vi "Get Objects in Range.vi"(8 "error in":errorcluster, 9 "Upper Bound":u16 format="%.0x", 10 "Lower Bound":u16 format="%.0x", 11 "Sorted Object Dictionary in":refnum<class "Sorted Object Dictionary.lvclass">) -> (0 "error out":errorcluster, 2 "Entries":refnum<class "OD Entry.lvclass">[](array[class]), 3 "Sorted Object Dictionary out":refnum<class "Sorted Object Dictionary.lvclass">)   [LabVIEW 2019, in "Electronic Datasheet.lvlib" / "Sorted Object Dictionary.lvclass"]
uses:
  Sorted Object Dictionary.lvclass
  OD Entry/OD Entry.lvclass
  Sorted Object Dictionary.lvclass/Sorted Object Dictionary.ctl
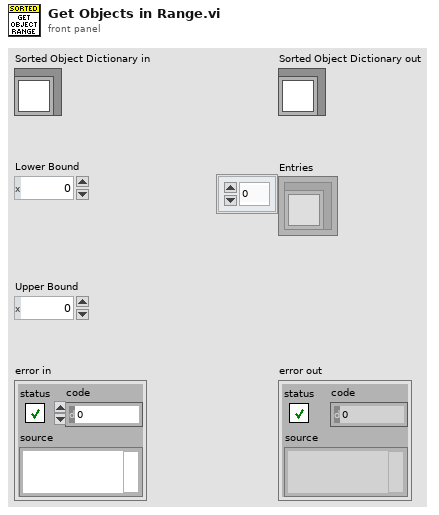
[diagram p1: front panel]
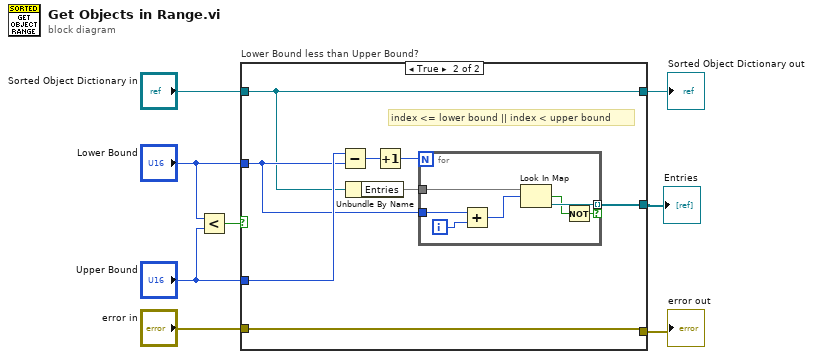
[diagram p0: block diagram]
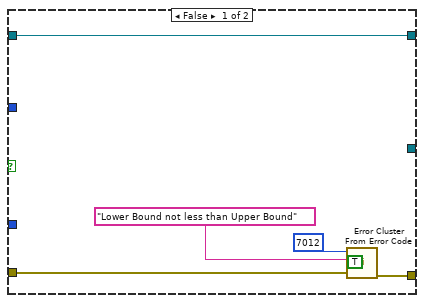
[diagram p2: hidden frame]
diagram:
  n1 = Less?(x="Lower Bound", y="Upper Bound") -> (x < y?=w5:bool)
  n2 = case "Lower Bound less than Upper Bound?" shown="True" w5 {
    tunnel: "Sorted Object Dictionary in" -> [w9 w16]
    tunnel: "Lower Bound" -> [_ w18]
    tunnel: "Upper Bound" -> [_ w21]
    tunnel: "error in" -> [w14 w17]
    tunnel: [w13 w17] -> w3
    tunnel: [w9 w16] -> w2
    tunnel: [_ w15] -> w1
    frame False {
      n3 = call <vilib>:"Error Cluster From Error Code.vi"("show call chain? (False)"=TRUE, "error in (no error)"=w14, "error message (\"\")"="Lower Bound not less than Upper Bound" ("error message (\"\")"), "error code (0)"=7012) -> ("error out"=w13:errorcluster)  [unwired: 5 in]
    }
    frame True {
      # "index <= lower bound || index < upper bound"
      n4 = Subtract(x=w21, y=w18) -> (x-y=w22:u16)
      n5 = Unbundle By Name(w16) -> ("Entries"=w19:map{u16, refnum<class "OD Entry.lvclass">})
      n6 = Increment(x=w22) -> (x+1=w20:u16)
      n7 = for {
        N: w20 -> [_]
        tunnel: w19 -> [w29]
        tunnel: w18 -> [w28]
        tunnel: [w25] -> w15 mode=indexing if=w23
        i -> [w26]
        n8 = Add(x=w28, y=w26) -> (x+y=w27:i32)
        n9 = Look In Map(map=w29, key=w27) -> (key not found?=w24:bool, value=w25:refnum<class "OD Entry.lvclass">)  [unwired: 1 in]
        n10 = Not(x=w24) -> (.not. x?=w23:bool)
      }
    }
  }
  "error out" <- w3
  "Sorted Object Dictionary out" <- w2
  "Entries" <- w1
